vi "ADIS16448 Read Register.vi"(8 "error in (no error)":errorcluster, 10 "ADIS16448 Register":T1 items=["Reserved1"=0, "DIAG_STAT"=2, "X_GYRO_LOW"=4, "X_GYRO_OUT"=6, "Y_GYRO_LOW"=8, "Y_GYRO_OUT"=10, "Z_GYRO_LOW"=12, "Z_GYRO_OUT"=14, "X_ACCL_LOW"=16, "X_ACCL_OUT"=18, "Y_ACCL_LOW"=20, "Y_ACCL_OUT"=22, "Z_ACCL_LOW"=24, "Z_ACCL_OUT"=26, "TEMP_OUT"=28, "TIME_STAMP"=30, "Reseved2"=32, "DATA_CNTR"=34, "X_DELTANG_LOW"=36, "X_DELTANG_OUT"=38, "Y_DELTANG_LOW"=40, "Y_DELTANG_OUT"=42, "Z_DELTANG_LOW"=44, "Z_DELTANG_OUT"=46, "X_DELTVEL_LOW"=48, "X_DELTVEL_OUT"=50, "Y_DELTVEL_LOW"=52, "Y_DELTVEL_OUT"=54, "Z_DELTVEL_LOW"=56, "Z_DELTVEL_OUT"=58, "Reserved3"=60, "Reserved4"=62, "XG_BIAS_LOW"=64, "XG_BIAS_HIGH"=66, "YG_BIAS_LOW"=68, "YG_BIAS_OUT"=70, "ZG_BIAS_LOW"=72, "ZG_BIAS_OUT"=74, "XA_BIAS_LOW"=76, "XA_BIAS_HIGH"=78, "YA_BIAS_LOW"=80, "YA_BIAS_OUT"=82, "ZA_BIAS_LOW"=84, "ZA_BIAS_OUT"=86, "Reserved5"=88, "Reserved6"=90, "FILT_CTRL"=92, "Reserved5"=94, "MSC_CTRL"=96, "UP_SCALE"=98, "DEC_RATE"=100], 11 "SPIDevRef in":T2) -> (0 "error out":errorcluster, 2 "Register Value":u16, 3 "SPIDevRef out":T2)   [LabVIEW 2025]
uses:
  <vilib>/Rock Robotics/WPI/SPI/WPI_SPIDevRef.ctl
  <vilib>/Rock Robotics/SystemInterfaces/spilib/spi_bus.ctl
  <vilib>/Rock Robotics/WPI/ThirdParty/ADI/ADIS16448/Typedef/ADIS16448 Register.ctl
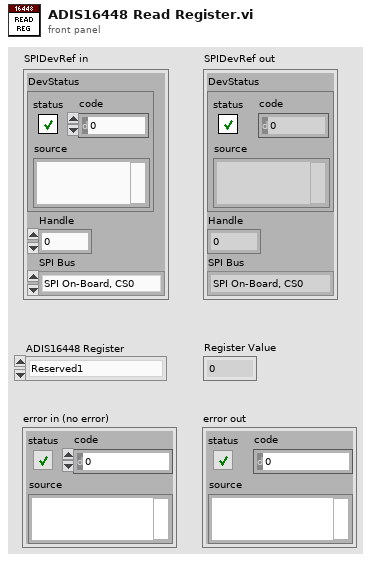
[diagram p1: front panel]
types:
  T1 = typedef "ADIS16448 Register.ctl" = u8
  T2 = typedef "WPI_SPIDevRef.ctl" = cluster{"DevStatus":errorcluster, "Handle":i32, "SPI Bus":T3}
  T3 = typedef "spi_bus.ctl" = enum16{"SPI On-Board, CS0", "SPI On-Board, CS1", "SPI On-Board, CS2", "SPI On-Board, CS3", "SPI MXP", "Invalid"}
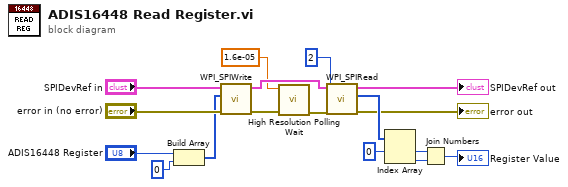
[diagram p0: block diagram]
diagram:
  n1 = Build Array("ADIS16448 Register", u8 0 ("element")) -> (w10:T1[])
  n2 = call <vilib>:"WPI_SPIWrite.vi"("error in (no error)"="error in (no error)", "Data To Send"=w10, "SPIDevRef"="SPIDevRef in") -> ("error out"=w5:errorcluster, "SPIDevRef"=w3:T2)  [unwired: 7 out]
  n3 = call <vilib>:"High Resolution Polling Wait.vi"("error in (no error)"=w5, "seconds to wait"=1.6e-05) -> ("error out"=w4:errorcluster)  [unwired: 9 in]
  n4 = call <vilib>:"WPI_SPIRead.vi"("error in (no error)"=w4, "Num to Read"=2, "SPIDevRef"=w3) -> ("error out"=→"error out":errorcluster, "Received Data"=w12:u8[], "SPIDevRef"=→"SPIDevRef out":T2)  [unwired: 6 in]
  n5 = Index Array(array=w12, index #1=0 ("index")) -> (element #1=w9:u8, element #2=w8:u8)  [unwired: 1 in]
  n6 = Join Numbers(hi=w9, lo=w8) -> ((hi.lo)=→"Register Value":u16)
